vi "Z drift - measure and compensate.vi"() -> ()   [LabVIEW 2019]
doc: "This example records the Z channel (ie the tip height) and calculates the drift along this axis. The drift speed can then be applied to compensate for it.\nBefore starting the measurement, the tip must be in contact with the sample and the Z-Controller must be running.\n\n- Nanonis Programming Interface -"
uses:
  <userlib>/Nanonis Prog Interface V5/Nanonis Prog Interface.lvlib
  <vilib>/Analysis/NI_AALPro.lvlib
panel:
  in  "Compensate":bool
  out "Stop [internal]":bool
  out "oStart":refnum<k4>
  in  "Start":bool
  in  "Quit":bool
  out "AllQuit":bool=TRUE
  in  "stop":bool
  out "Drift (m/s)":dbl format="%#_4p"
  out "XY Graph":cluster{dbl[], "Best Linear Fit":dbl[]}[](graph)
  in  "Duration":dbl=60.0 format="%<%H:%M:%S>t"
  # "Example program for the Nanonis programming interface\n\n-  Measure the drift speed along Z -"
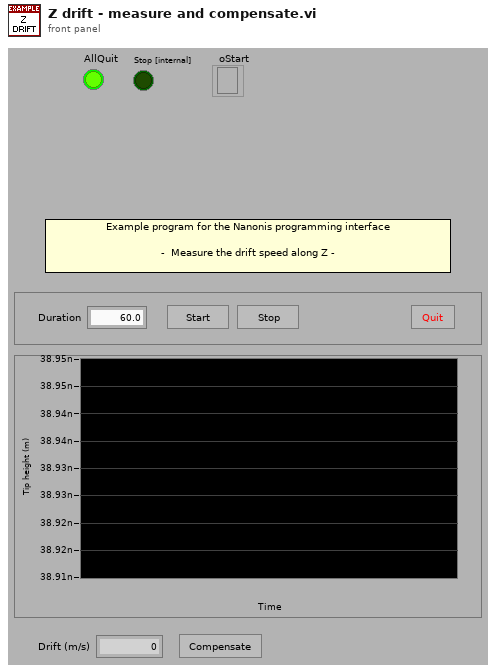
[diagram p1: front panel]
types:
  T1 = cluster{"Array":dbl[], "Best Linear Fit":dbl[]}[]
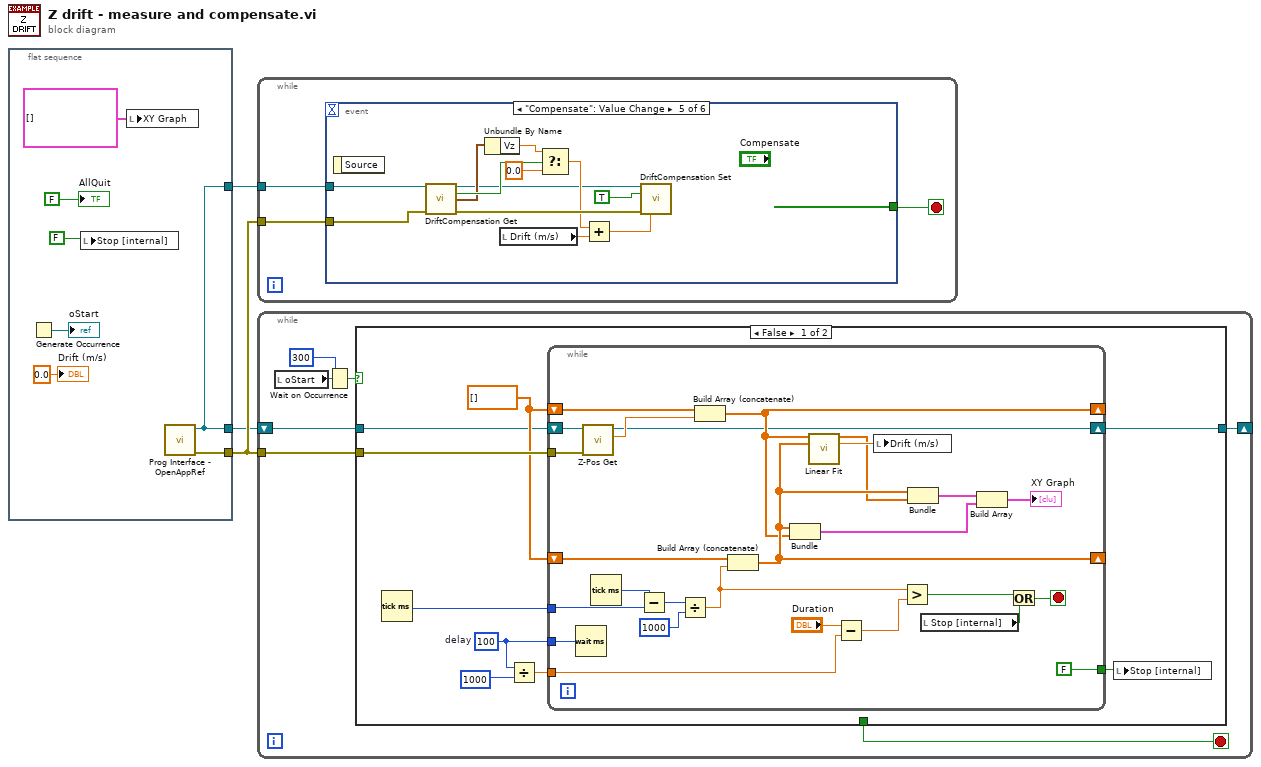
[diagram p0: block diagram]
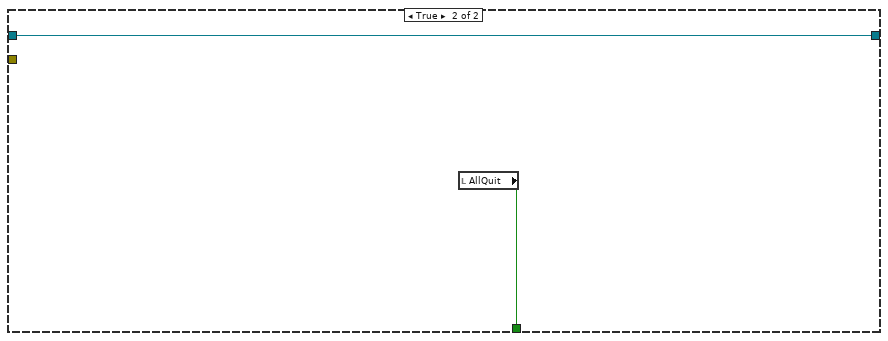
[diagram p2: hidden frame]
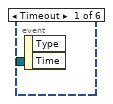
[diagram p3: hidden frame]
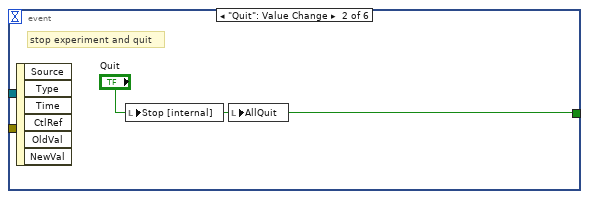
[diagram p4: hidden frame]
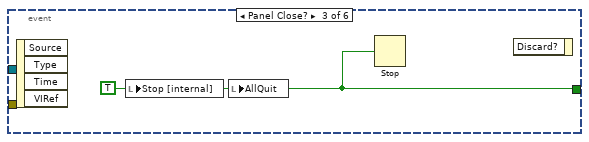
[diagram p5: hidden frame]
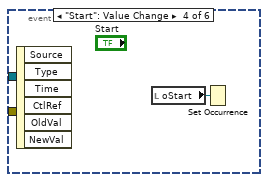
[diagram p6: hidden frame]
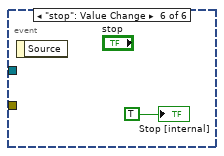
[diagram p7: hidden frame]
diagram:
  n1 = flat-sequence {
    tunnel: [w10] -> w3
    tunnel: [w4] -> w1
    tunnel: [w4] -> w2
    frame #0 {
      n2 = Generate Occurrence() -> (→"oStart":refnum<k4>)
      n3 = local write "Stop [internal]"(FALSE ("stop")) -> ()
      n4 = local write "XY Graph"(T1 [] ("XY Graph")) -> ()
      n5 = call <userlib>:"Prog Interface - OpenAppRef.vi"() -> ("Error out"=w10:errorcluster, "Application reference"=w4:refnum<vi>)  [unwired: 6 in]
      "Drift (m/s)" <- 0.0 ("Slope")
      "AllQuit" <- FALSE ("AllQuit")
    }
  }
  n6 = while {
    tunnel: w3 -> [w12]
    tunnel: w2 -> [w11]
    stop <- w13 stop-if-true
    n7 = event shown="[4] \"Compensate\": Value Change" {
      selector: _ -> [_ _ _ _ _ _]
      dyn-events: _ -> [_ _ _ _ _ _]
      timeout: _ -> [_ _ _ _ _ _]
      tunnel: [_ "Quit" w15 _ _ _] -> w13
      tunnel: w12 -> [_ _ _ _ w27 _]
      tunnel: w11 -> [_ _ _ _ w18 _]
      event Timeout {
        n8 = event-data() -> ()  [unwired: 1 in, 2 out]
      }
      event "Quit": Value Change {
        # "stop experiment and quit"
        n9 = event-data() -> ()  [unwired: 1 in, 6 out]
        n10 = local write "Stop [internal]"("Quit") -> ()
        n11 = local write "AllQuit"("Quit") -> ()
      }
      event Panel Close? {
        w15 = TRUE ("Quit")
        n12 = event-data() -> ()  [unwired: 1 in, 4 out]
        n13 = local write "Stop [internal]"(w15) -> ()
        n14 = local write "AllQuit"(w15) -> ()
        n15 = Stop(stop? (T)=w15) -> ()
        n16 = event-data() -> ()  [unwired: 2 in, 1 out]
      }
      event "Start": Value Change {
        n17 = event-data() -> ()  [unwired: 1 in, 6 out]
        n18 = local read "oStart"() -> (w16:refnum<k4>)
        n19 = Set Occurrence(w16) -> ()
      }
      event "Compensate": Value Change {
        n20 = event-data() -> ()  [unwired: 1 in, 1 out]
        n21 = call <userlib>:"DriftCompensation Get.vi"("Application ref in"=w18, "error in (no error)"=w27) -> ("Application ref out"=w17:refnum<vi>, "Compensation status"=w25:bool, "Compensation speeds (m/s)"=w24:cluster{"Vx":sgl, "Vy":sgl, "Vz":sgl}, "error out"=w26:errorcluster)  [unwired: 9 in, 1 out]
        n22 = Unbundle By Name(w24) -> ("Vz"=w23:sgl)
        n23 = local read "Drift (m/s)"() -> (w20:dbl)
        n24 = Select(t=w23, s=w25, f=sgl 0.0) -> (s? t:f=w21:sgl)
        n25 = Add(x=w21, y=w20) -> (x+y=w19:dbl)
        n26 = call <userlib>:"DriftCompensation Set.vi"("Application ref in"=w17, "Compensation On/Off"=TRUE, "error in (no error)"=w26, "Vz (m/s)"=w19) -> ()  [unwired: 10 in, 2 out]
      }
      event "stop": Value Change {
        n27 = event-data() -> ()  [unwired: 1 in, 1 out]
        "Stop [internal]" <- TRUE ("Stop [internal]")
      }
    }
  }
  n28 = while {
    tunnel: w3 -> [w36]
    shift-right: [w30] -> _
    shift-left: w1 -> [w31]
    stop <- w33 stop-if-true
    n29 = local read "oStart"() -> (w35:refnum<k4>)
    n30 = Wait on Occurrence(2:w35, 3:300 ("ms timeout (-1)")) -> (0:w34:bool)  [unwired: 1 in]
    n31 = case shown="False" w34 {
      tunnel: w36 -> [w45 _]
      tunnel: [_ w73] -> w33
      tunnel: w31 -> [w38 w72]
      tunnel: [w37 w72] -> w30
      frame False {
        w42 = u32 100  # delay
        w43 = sgl[] [] ("Array")
        n32 = Tick Count (ms)() -> (millisecond timer value=w44:u32)
        n33 = Divide(x=w42, y=u32 1000) -> (x/y=w40:dbl)
        n34 = while {
          tunnel: w45 -> [w71]
          shift-right: [w50] -> _
          shift-left: w43 -> [w69]
          shift-right: [w52] -> _
          shift-left: w43 -> [w68]
          tunnel: w44 -> [w67]
          tunnel: w42 -> [w55]
          tunnel: w40 -> [w54]
          tunnel: [FALSE] -> w39
          shift-right: [w46] -> w37
          shift-left: w38 -> [w47]
          stop <- w62 stop-if-true
          n35 = Wait (ms)(milliseconds to wait=w55) -> ()  [unwired: 1 out]
          n36 = call <userlib>:"Z-Pos Get.vi"("error in (no error)"=w71, "Application ref in"=w47) -> ("Z position (m)"=w70:sgl, "Application ref out"=w46:refnum<vi>)  [unwired: 7 in, 1 out]
          n37 = Tick Count (ms)() -> (millisecond timer value=w61:u32)
          n38 = Subtract(x=w61, y=w67) -> (x-y=w65:u32)
          n39 = Divide(x=w65, y=u32 1000) -> (x/y=w64:dbl)
          n40 = Build Array (concatenate)(w69, w70) -> (w50:sgl[])
          n41 = Build Array (concatenate)(w68, w64) -> (w52:dbl[])
          n42 = Bundle(w52, w50) -> (w58:cluster{dbl[], sgl[]})  [unwired: 1 in]
          n43 = call <vilib>:"Linear Fit.vi"("Y"=w50, "X"=w52) -> ("Best Linear Fit"=w49:dbl[], "slope"=w51:dbl)  [unwired: 9 in, 3 out]
          n44 = Subtract(x="Duration", y=w54) -> (x-y=w60:dbl)
          n45 = local write "Drift (m/s)"(w51) -> ()
          n46 = Greater?(x=w64, y=w60) -> (0:w63:bool)
          n47 = Bundle(w52, "Best Linear Fit"=w49) -> (w53:cluster{dbl[], "Best Linear Fit":dbl[]})  [unwired: 1 in]
          n48 = local read "Stop [internal]"() -> (w57:bool)
          n49 = Build Array(w53, w58) -> (→"XY Graph":cluster{dbl[], "Best Linear Fit":dbl[]}[])
          n50 = Or(x=w63, y=w57) -> (x .or. y?=w62:bool)
        }
        n51 = local write "Stop [internal]"(w39) -> ()
      }
      frame True {
        n52 = local read "AllQuit"() -> (w73:bool)
      }
    }
  }
